vi "XY Graph Special Event Handler Wrapper.vi"(8 "Error In":errorcluster, 11 "XY Graph Event":T1) -> (0 "Error Out":errorcluster, 3 "Message":string)   [LabVIEW 2021, in "XY Graph Add-Ons.lvlib"]
uses:
  XY Graph Add-Ons.lvlib
  XY Graph Event.ctl
  <vilib>/Utility/miscctls.llb/LVPoint32TypeDef.ctl
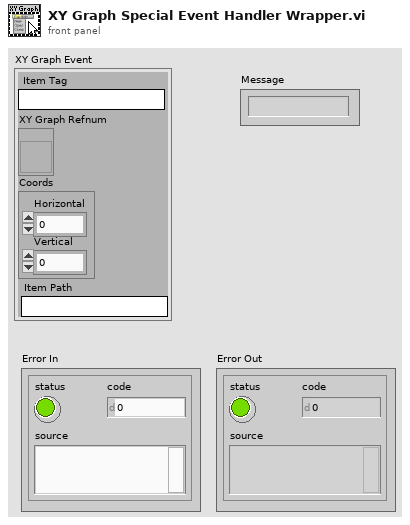
[diagram p1: front panel]
types:
  T1 = typedef "XY Graph Add-Ons.lvlib/XY Graph Event.ctl" = cluster{"Item Tag":string, "XY Graph Refnum":refnum<vi>, "Coords":T2, "Item Path":string}
  T2 = typedef "LVPoint32TypeDef.ctl" = cluster{"Horizontal":i32, "Vertical":i32}
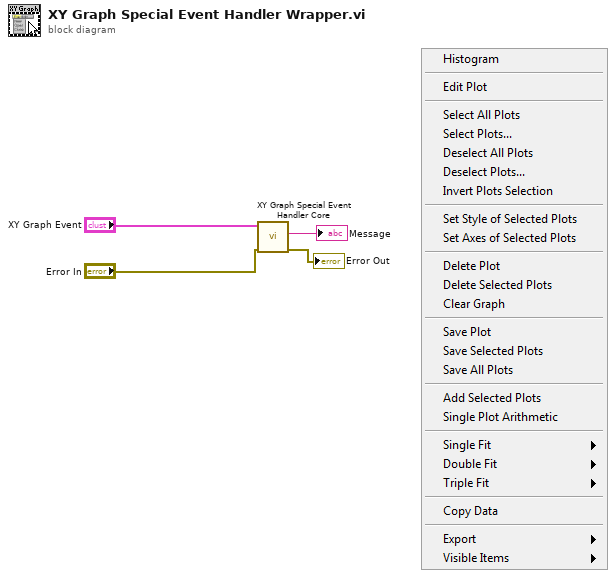
[diagram p0: block diagram]
diagram:
  n1 = call "XY Graph Special Event Handler Core.vi"("error in (no error)"="Error In", "XY Graph Event"="XY Graph Event") -> ("error out"=→"Error Out":errorcluster, "Message"=→"Message":string)  [unwired: 5 in, 3 out]
